vi "Get position 2.vi"(5 "Motor params":T1={"Action"=2, "Direction motor 1"=1, "Direction motor 2"=1, "Steps motor 1"=100, "Steps motor 2"=100, "Step style motor 1"=1, "Step style motor 2"=1} {"Step style motor 2" items=["", "Single", "Double", "Interleave", "Microstep"]; "Step style motor 1" items=["", "Single", "Double", "Interleave", "Microstep"]; "Direction motor 2" items=["", "Forward", "Backward"]; "Direction motor 1" items=["", "Forward", "Backward"]; "Action" items=["", "Initialize", "Move"]}, 7 "°/step":dbl[](array[numeric])=[0.01, 0.01], 8 "error in (no error)":errorcluster, 10 "Positions in":dbl[](array[numeric]), 11 "VISA resource name in":refnum<visa-resource-name>) -> (0 "error out":errorcluster, 2 "Positions out":dbl[](array[numeric]), 3 "VISA Refnum out":refnum<visa-resource-name>)   [LabVIEW 2020, in "Control de MaP.lvlib"]
uses:
  Control de MaP.lvlib
  Controls/Move motor parameters--cluster.ctl
  Controls/Motor direction.ctl
  Controls/Step style.ctl
  Write--command.vi
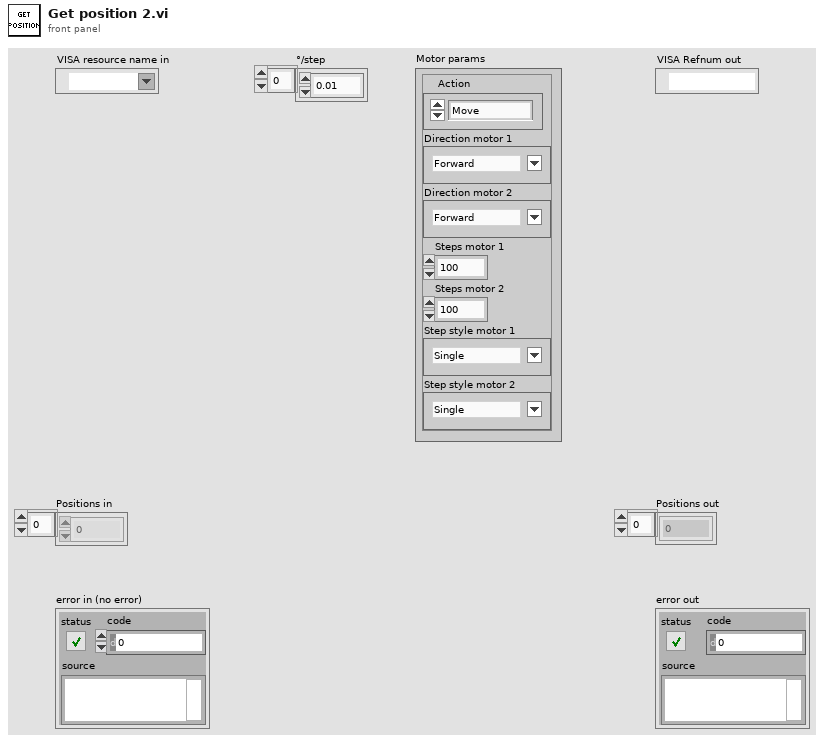
[diagram p1: front panel]
types:
  T1 = typedef "Control de MaP.lvlib/Move motor parameters--cluster.ctl" = cluster{"Action":u8, "Direction motor 1":T2, "Direction motor 2":T2, "Steps motor 1":u16, "Steps motor 2":u16, "Step style motor 1":T3, "Step style motor 2":T3}
  T2 = typedef "Control de MaP.lvlib/Motor direction.ctl" = u8
  T3 = typedef "Control de MaP.lvlib/Step style.ctl" = u8
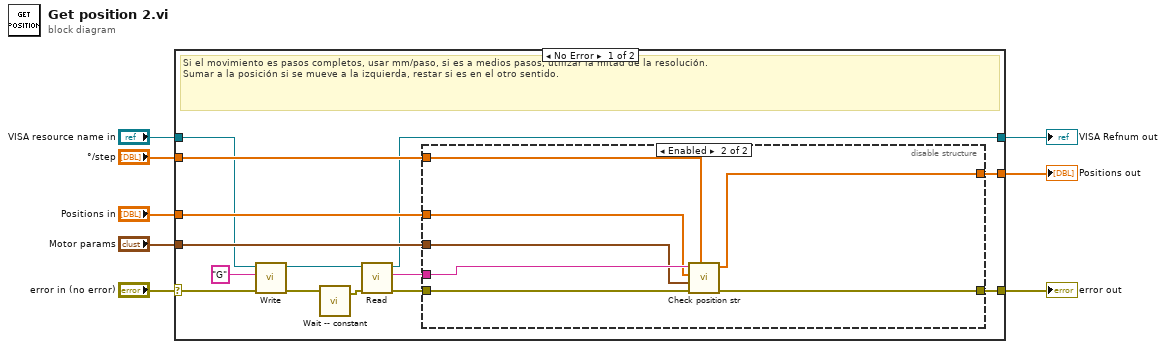
[diagram p0: block diagram]
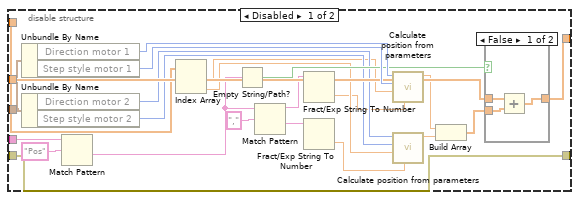
[diagram p2: hidden frame]
diagram:
  n1 = case shown="No Error" "error in (no error)" {
    selector: "error in (no error)" -> [w15 w57]
    tunnel: [w22 w59] -> w8
    tunnel: "Positions in" -> [w21 w59]
    tunnel: [w10 w57] -> w7
    tunnel: "Motor params" -> [w20 _]
    tunnel: "°/step" -> [w19 _]
    tunnel: "VISA resource name in" -> [w13 w58]
    tunnel: [w11 w58] -> w1
    frame No Error {
      # "Si el movimiento es pasos completos, usar mm/paso, si es a medios pasos, utilizar la mitad de la resolución.\nSumar a la posición si se mueve a la izquierda, restar si es en el otro sentido."
      n2 = call-poly "Write.vi"("error in (no error)"=w15, "Command"="G", "VISA resource name"=w13) -> ("error out"=w17:errorcluster, "VISA resource name out"=w18:refnum<visa-resource-name>)  [unwired: 6 in, 1 out]
      n3 = call "Wait -- constant.vi"("error in (no error)"=w17) -> ("error out"=w16:errorcluster)  [unwired: 4 in]
      n4 = call "Read.vi"("error in (no error)"=w16, "VISA resource name"=w18) -> ("error out"=w9:errorcluster, "Recibo de Datos"=w12:string, "VISA resource name out"=w11:refnum<visa-resource-name>)  [unwired: 6 in, 1 out]
      n5 = disable-structure shown="Enabled" {
        disable-tunnel: [w42 w55] -> w22
        disable-tunnel: w21 -> [w41 w51]
        disable-tunnel: w20 -> [w39 w50]
        disable-tunnel: w19 -> [w36 w56]
        disable-tunnel: w12 -> [w24 w52]
        disable-tunnel: w9 -> [w23 w54]
        disable-tunnel: [w23 w53] -> w10
        frame Disabled {
          n6 = Unbundle By Name(w39) -> ("Direction motor 1"=w43:T2, "Step style motor 1"=w44:T3)
          n7 = Unbundle By Name(w39) -> ("Direction motor 2"=w37:T2, "Step style motor 2"=w38:T3)
          n8 = Match Pattern(string=w24, regular expression="Pos") -> (after substring=w29:string)  [unwired: 1 in, 3 out]
          n9 = Index Array(array=w36) -> (element #1=w35:dbl, element #2=w34:dbl)  [unwired: 2 in]
          n10 = Empty String/Path?(string/path=w29) -> (empty?=w40:bool)
          n11 = Match Pattern(string=w29, regular expression=",") -> (before substring=w25:string, after substring=w27:string)  [unwired: 1 in, 2 out]
          n12 = Fract/Exp String To Number(string=w25) -> (number=w30:dbl)  [unwired: 3 in, 1 out]
          n13 = Fract/Exp String To Number(string=w27) -> (number=w26:dbl)  [unwired: 3 in, 1 out]
          n14 = call "Calculate position from parameters.vi"("Current step"=w30, "°/step"=w35, "Step style motor"=w44, "Motor direction"=w43) -> ("Position adjustment"=w32:dbl)  [unwired: 6 in, 1 out]
          n15 = call "Calculate position from parameters.vi"("Current step"=w26, "°/step"=w34, "Step style motor"=w38, "Motor direction"=w37) -> ("Position adjustment"=w31:dbl)  [unwired: 6 in, 1 out]
          n16 = Build Array(w32, w31) -> (w33:dbl[])
          n17 = case shown="False" w40 {
            tunnel: [w48 w49] -> w42
            tunnel: w33 -> [w47 _]
            tunnel: w41 -> [w46 w49]
            frame False {
              n18 = Add(x=w46, y=w47) -> (x+y=w48:dbl[])
            }
            frame True {
            }
          }
        }
        frame Enabled {
          n19 = call "Check position str.vi"("°/step"=w56, "error in (no error)"=w54, "Motor params"=w50, "Positions"=w51, "Recibo de Datos"=w52) -> ("error out"=w53:errorcluster, "Positions out"=w55:dbl[])  [unwired: 5 in]
        }
      }
    }
    frame Error {
    }
  }
  "Positions out" <- w8
  "error out" <- w7
  "VISA Refnum out" <- w1
